vi "Check if Package Exists in Feed.vi"(8 "error in":errorcluster, 10 "package filename":string, 11 "feed folderpath in":path) -> (0 "error out":errorcluster, 2 "package exists?":bool, 3 "feed folderpath out":path)   [LabVIEW 2014, in "NIPM_API.lvlib"]
doc: "Checks whether a package exists in a feed\n\nINPUT(s)\n<B>Feed folderpath</B>: Specifies the folder containing the feed\n\n<B>Package filename</B>: Specifies the package filename that this VI will look for in the specified feed folderpath\n\nOUTPUT(s)\n<B>Feed folderpath out</B>: Outputs the specified feed folderpath\n\n<B>Package exists?</B>: Outputs whether or not the specified package exists in the specified feed"
uses:
  NIPM_API.lvlib
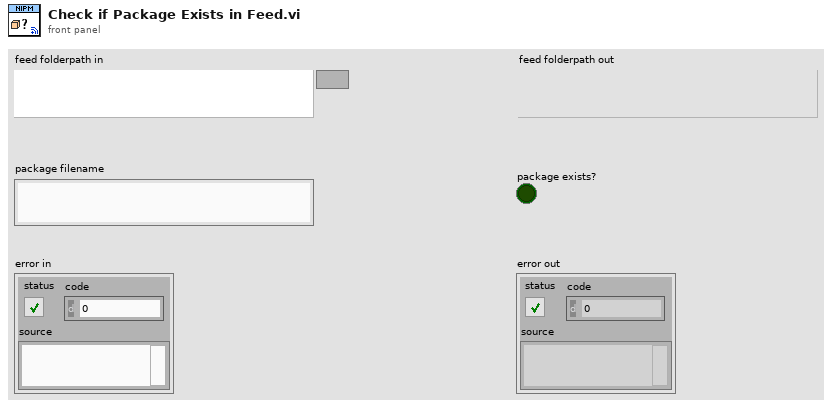
[diagram p1: front panel]
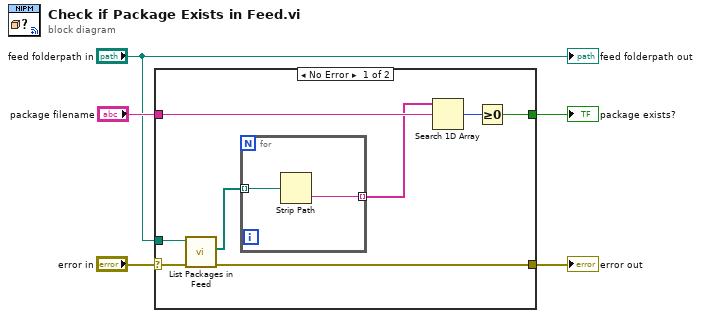
[diagram p0: block diagram]
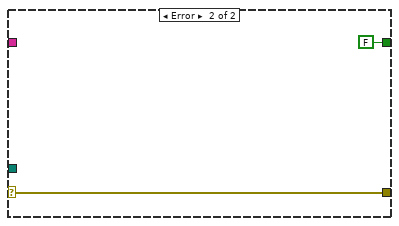
[diagram p2: hidden frame]
diagram:
  n1 = case shown="No Error" "error in" {
    selector: "error in" -> [w12 w17]
    tunnel: "feed folderpath in" -> [w13 _]
    tunnel: "package filename" -> [w11 _]
    tunnel: [w10 w17] -> w3
    tunnel: [w8 FALSE] -> w2
    frame No Error {
      n2 = call "List Packages in Feed.vi"("error in"=w12, "feed folderpath in"=w13) -> ("error out"=w10:errorcluster, "package relative filepaths"=w7:path[])  [unwired: 6 in, 2 out]
      n3 = for {
        tunnel: w7 -> [w15] mode=indexing
        tunnel: [w14] -> w6 mode=indexing
        n4 = Strip Path(path=w15) -> (name=w14:string)  [unwired: 1 out]
      }
      n5 = Search 1D Array(1D array=w6, element=w11) -> (index of element=w9:i32)  [unwired: 1 in]
      n6 = Greater Or Equal To 0?(x=w9) -> (x >= 0?=w8:bool)
    }
    frame Error {
    }
  }
  "error out" <- w3
  "package exists?" <- w2
  "feed folderpath out" <- "feed folderpath in"
